vi "girpcutil_GetRpcValue.vi"(8 "Fehler (Eingang, kein Fehler)":errorcluster, 9 "member":string, 10 "value":i32, 11 "girpcutil_params":T1) -> (0 "Fehler (Ausgang)":errorcluster, 2 "result":i32)   [LabVIEW 2016]
uses:
  girpcutil_params.ctl
panel:
  out "errMsg 2":u8[](array[numeric])
  out "errMsgLen 2":i32
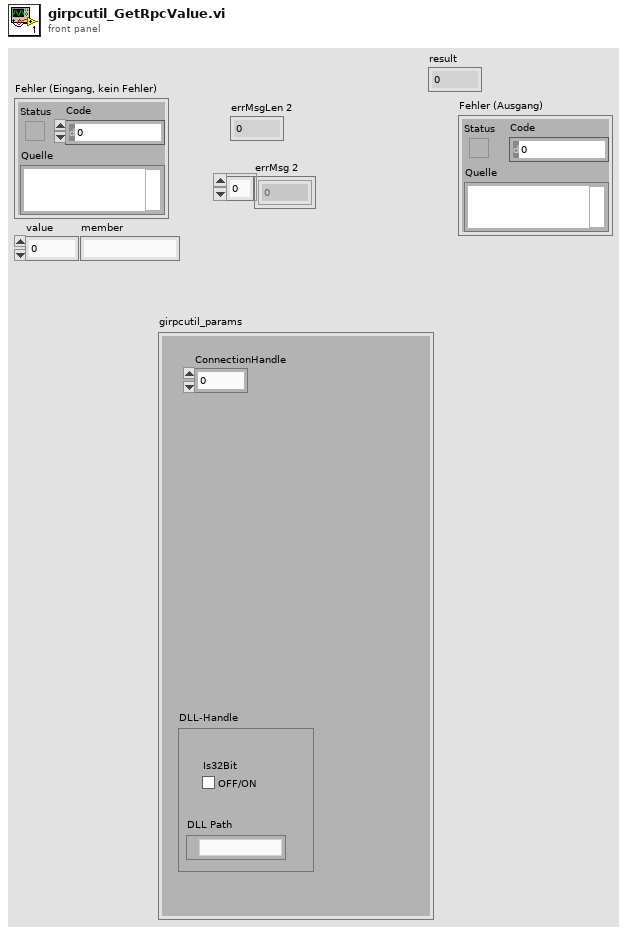
[diagram p1: front panel]
types:
  T1 = typedef "girpcutil_params.ctl" = cluster{"ConnectionHandle":i32, "DLL-Handle":cluster{"DLL Path":path, "Is32Bit":bool}}
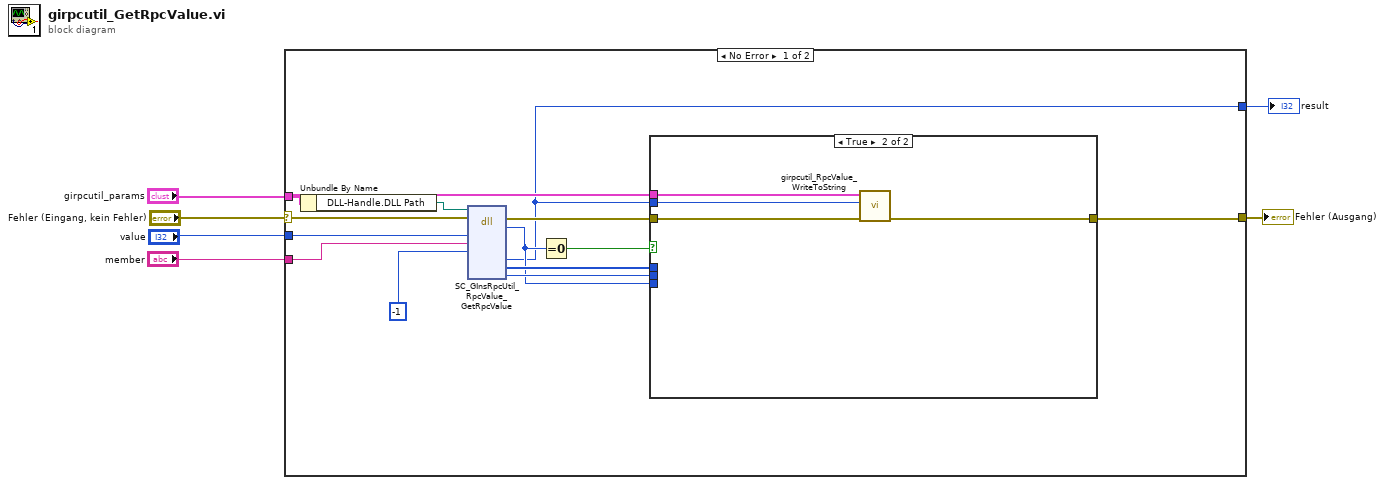
[diagram p0: block diagram]
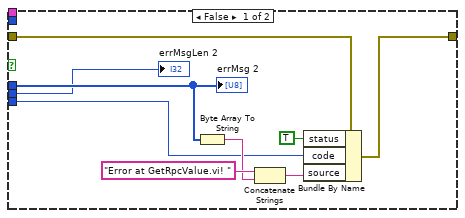
[diagram p2: hidden frame]
diagram:
  n1 = case shown="No Error" "Fehler (Eingang, kein Fehler)" {
    selector: "Fehler (Eingang, kein Fehler)" -> [w19 w33]
    tunnel: [w11 w33] -> w5
    tunnel: "girpcutil_params" -> [w12 _]
    tunnel: "value" -> [w17 _]
    tunnel: "member" -> [w16 _]
    tunnel: [w7 _] -> w1
    frame No Error {
      n2 = Unbundle By Name(w12) -> ("DLL-Handle.DLL Path"=w18:path)
      n3 = dll-call lib="?" fn="SC_GInsRpcUtil_RpcValue_GetRpcValue"(path in=w18, error in=w19, "value"=w17, "member"=w16, "index"=-1) -> (error out=w14:errorcluster, "Rückgabewert"=w8:i32, "result"=w7:i32, "errMsg"=w9:u8[], "errMsgLen"=w10:i32)  [unwired: 7 in, 1 out]
      n4 = Equal To 0?(x=w8) -> (x = 0?=w13:bool)
      n5 = case shown="True" w13 {
        tunnel: w14 -> [w22 w32]
        tunnel: [w21 w31] -> w11
        tunnel: w9 -> [w26 _]
        tunnel: w10 -> [w23 _]
        tunnel: w8 -> [w20 _]
        tunnel: w7 -> [_ w30]
        tunnel: w12 -> [_ w29]
        frame False {
          n6 = Byte Array To String(unsigned byte array=w26) -> (string=w27:string)
          n7 = Concatenate Strings("Error at GetRpcValue.vi! " ("source"), w27) -> (w25:string)
          n8 = Bundle By Name(cluster=w22, "status"=TRUE, "code"=w20, "source"=w25) -> (w21:errorcluster)
          "errMsg 2" <- w26
          "errMsgLen 2" <- w23
        }
        frame True {
          n9 = call "girpcutil_RpcValue_WriteToString.vi"("Fehler (Eingang, kein Fehler)"=w32, "value"=w30, "girpcutil_params"=w29) -> ("Fehler (Ausgang)"=w31:errorcluster)  [unwired: 8 in]
        }
      }
    }
    frame Error {
    }
  }
  "Fehler (Ausgang)" <- w5
  "result" <- w1
